vi "WriteNewCarexFile.vi"(6 "Overwrite?(F)":bool, 8 "error in (no error)":errorcluster, 9 "Proposed File Name":string, 10 "Output Path":path, 11 "CarexData In":refnum<class "CAlexData.lvclass">) -> (0 "error out":errorcluster, 1 "Actual File Name":string, 3 "CarexData Out":refnum<class "CAlexData.lvclass">)   [LabVIEW 2014, in "CAlexData.lvclass"]
uses:
  CAlexData.lvclass
  <vilib>/Utility/file.llb/Write To Spreadsheet File (string).vi
  LabView/CustomVI/CustomVI.lvlib
panel:
  out "ATIsensor":dbl[][](array[numeric])
  out "ForceComp":dbl[][](array[numeric])
  out "FieldForce":dbl[][](array[numeric])
  out "ShoulderCenter":dbl[][](array[numeric])
  out "CableLength":dbl[][](array[numeric])
  out "WaistPosition":dbl[][](array[numeric])
  out "CableTension":dbl[][](array[numeric])
  out "RefTension":dbl[][](array[numeric])
  out "JointAngle":dbl[][](array[numeric])
  out "Marker":string[](array[string])
  out "Time":dbl[](array[numeric])
  out "ExpCondition":T1
  out "ArmLength":cluster{"Upper":dbl, "Lower":dbl}
  out "FFG":T2
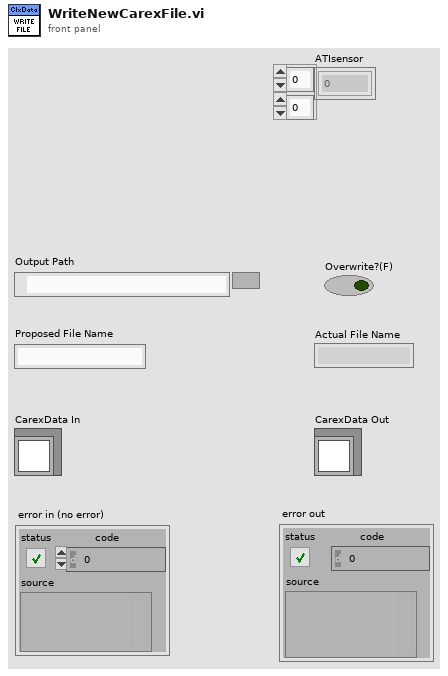
[diagram p1: front panel]
types:
  T1 = cluster{"MotorOn":bool, "EstGH":bool, "TensionMode":u16}
  T2 = cluster{"Kn":dbl, "Ns":dbl, "Kt":dbl, "Kd":dbl, "Dn":dbl, "Dt":dbl}
  T3 = enum16{"open", "replace", "create", "open or create", "replace or create", "replace or create with confirmation"}
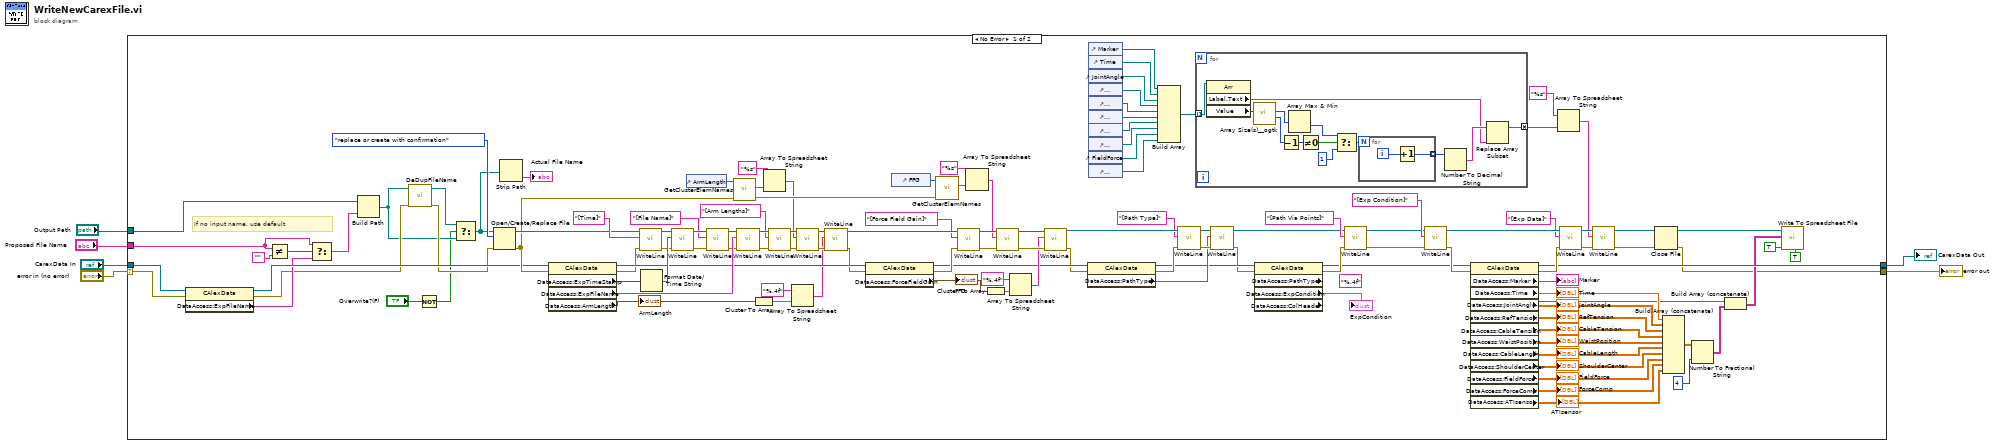
[diagram p0: block diagram]
diagram:
  n1 = case shown="No Error" "error in (no error)" {
    selector: "error in (no error)" -> [w68 w148]
    tunnel: [w73 w147] -> w5
    tunnel: [w10 w148] -> w6
    tunnel: "Output Path" -> [w60 _]
    tunnel: "CarexData In" -> [w69 w147]
    tunnel: "Proposed File Name" -> [w65 _]
    frame No Error {
      (unwired) "%.4f" ("format string")
      # "If no input name, use default"
      n2 = property class="CAlexData"(reference=w69, error in=w68) -> (reference out=w67:refnum<class "CAlexData.lvclass">, error out=w58:errorcluster, "DataAccess:ExpFileName"=w64:string)
      n3 = Not Equal?(x=w65, y="") -> (x != y?=w66:bool)
      n4 = Select(t=w65, s=w66, f=w64) -> (s? t:f=w59:string)
      n5 = Build Path(base path=w60, name or relative path=w59) -> (appended path=w56:path)
      n6 = call "DeDupFileName.vi"("error in (no error)"=w58, "Path"=w56) -> ("error out"=w57:errorcluster, "Out Path"=w63:path)  [unwired: 8 in]
      n7 = Not(x="Overwrite?(F)") -> (.not. x?=w46:bool)
      n8 = Select(t=w63, s=w46, f=w56) -> (s? t:f=w15:path)
      n9 = Open/Create/Replace File(file path (use dialog)=w15, error in=w57, operation (0:open)=T3."replace or create with confirmation") -> (refnum out=w72:refnum<file>, error out=w71:errorcluster)  [unwired: 3 in, 1 out]
      n10 = Strip Path(path=w15) -> (name=→"Actual File Name":string)  [unwired: 1 out]
      n11 = property class="CAlexData"(reference=w67, error in=w71) -> (reference out=w118:refnum<class "CAlexData.lvclass">, error out=w87:errorcluster, "DataAccess:ExpTimeStamp"=w131:timestamp, "DataAccess:ExpFileName"=w129:string, "DataAccess:ArmLength"=w119:cluster{"Upper":dbl, "Lower":dbl})
      "ArmLength" <- w119
      n12 = call "WriteLine.vi"("error in (no error)"=w87, "text"="[Time]", "refnum in"=w72) -> ("error out"=w88:errorcluster, "refnum out"=w89:refnum<file>)  [unwired: 6 in, 1 out]
      n13 = Format Date/Time String(seconds (now)=w131) -> (date/time string=w130:string)  [unwired: 2 in]
      n14 = call "WriteLine.vi"("error in (no error)"=w88, "text"=w130, "refnum in"=w89) -> ("error out"=w85:errorcluster, "refnum out"=w84:refnum<file>)  [unwired: 6 in, 1 out]
      n15 = control-ref of="ArmLength"() -> (w54:refnum<vi>)
      n16 = call "WriteLine.vi"("error in (no error)"=w85, "text"="[File Name]", "refnum in"=w84) -> ("error out"=w83:errorcluster, "refnum out"=w82:refnum<file>)  [unwired: 6 in, 1 out]
      n17 = call "GetClusterElemNames.vi"("error in (no error)"=w71, "Cluster in"=w54) -> ("error out"=w55:errorcluster, "Element Names"=w50:string[])  [unwired: 6 in, 2 out]
      n18 = call "WriteLine.vi"("error in (no error)"=w83, "text"=w129, "refnum in"=w82) -> ("error out"=w128:errorcluster, "refnum out"=w127:refnum<file>)  [unwired: 6 in, 1 out]
      n19 = Cluster To Array(cluster=w119) -> (array=w126:dbl[])
      n20 = Array To Spreadsheet String(array=w50, 3:"%s" ("format string")) -> (spreadsheet string=w49:string)  [unwired: 1 in]
      n21 = call "WriteLine.vi"("error in (no error)"=w128, "text"="[Arm Lengths]", "refnum in"=w127) -> ("error out"=w124:errorcluster, "refnum out"=w123:refnum<file>)  [unwired: 6 in, 1 out]
      n22 = Array To Spreadsheet String(array=w126, 3:"%.4f" ("format string")) -> (spreadsheet string=w117:string)  [unwired: 1 in]
      n23 = call "WriteLine.vi"("error in (no error)"=w124, "text"=w49, "refnum in"=w123) -> ("error out"=w120:errorcluster, "refnum out"=w121:refnum<file>)  [unwired: 6 in, 1 out]
      n24 = call "WriteLine.vi"("error in (no error)"=w120, "text"=w117, "refnum in"=w121) -> ("error out"=w116:errorcluster, "refnum out"=w122:refnum<file>)  [unwired: 6 in, 1 out]
      n25 = property class="CAlexData"(reference=w118, error in=w116) -> (reference out=w104:refnum<class "CAlexData.lvclass">, error out=w113:errorcluster, "DataAccess:ForceFieldGain"=w110:T2)
      "FFG" <- w110
      n26 = control-ref of="FFG"() -> (w53:refnum<vi>)
      n27 = call "GetClusterElemNames.vi"("error in (no error)"=w55, "Cluster in"=w53) -> ("Element Names"=w52:string[])  [unwired: 6 in, 3 out]
      n28 = call "WriteLine.vi"("error in (no error)"=w113, "text"="[Force Field Gain]", "refnum in"=w122) -> ("error out"=w109:errorcluster, "refnum out"=w108:refnum<file>)  [unwired: 6 in, 1 out]
      n29 = Array To Spreadsheet String(array=w52, 3:"%s" ("format string")) -> (spreadsheet string=w51:string)  [unwired: 1 in]
      n30 = Cluster To Array(cluster=w110) -> (array=w111:dbl[])
      n31 = call "WriteLine.vi"("error in (no error)"=w109, "text"=w51, "refnum in"=w108) -> ("error out"=w107:errorcluster, "refnum out"=w106:refnum<file>)  [unwired: 6 in, 1 out]
      n32 = Array To Spreadsheet String(array=w111, 3:"%.4f" ("format string")) -> (spreadsheet string=w105:string)  [unwired: 1 in]
      n33 = call "WriteLine.vi"("error in (no error)"=w107, "text"=w105, "refnum in"=w106) -> ("error out"=w103:errorcluster, "refnum out"=w102:refnum<file>)  [unwired: 6 in, 1 out]
      n34 = property class="CAlexData"(reference=w104, error in=w103) -> (reference out=w93:refnum<class "CAlexData.lvclass">, error out=w101:errorcluster, "DataAccess:PathType"=w98:string)
      n35 = control-ref of="Marker"() -> (w43:refnum<vi>)
      n36 = control-ref of="Time"() -> (w42:refnum<vi>)
      n37 = control-ref of="JointAngle"() -> (w41:refnum<vi>)
      n38 = control-ref of="RefTension"() -> (w40:refnum<vi>)
      n39 = control-ref of="CableTension"() -> (w39:refnum<vi>)
      n40 = control-ref of="WaistPosition"() -> (w38:refnum<vi>)
      n41 = control-ref of="CableLength"() -> (w37:refnum<vi>)
      n42 = control-ref of="ShoulderCenter"() -> (w36:refnum<vi>)
      n43 = control-ref of="FieldForce"() -> (w35:refnum<vi>)
      n44 = control-ref of="ForceComp"() -> (w34:refnum<vi>)
      n45 = Build Array(w43, w42, w41, w40, w39, w38, w37, w36, w35, w34) -> (w33:refnum<vi>[])
      n46 = call "WriteLine.vi"("error in (no error)"=w101, "text"="[Path Type]", "refnum in"=w102) -> ("error out"=w100:errorcluster, "refnum out"=w99:refnum<file>)  [unwired: 6 in, 1 out]
      n47 = for {
        tunnel: w33 -> [w144] mode=indexing
        tunnel: [w140] -> w17 mode=concatenating
        n48 = property class="Arr"(reference=w144) -> ("Label.Text"=w141:string, "Value"=w139:variant)  [unwired: 1 in, 2 out]
        n49 = call <userlib>:"Array Size(s)__ogtk.vi"("Array"=w139) -> ("N dims"=w137:u32, "Size(s)"=w138:u32[])  [unwired: 8 in, 1 out]
        n50 = Decrement(x=w137) -> (x-1=w136:u32)
        n51 = Array Max & Min(array=w138) -> (min value=w132:u32)  [unwired: 3 out]
        n52 = Not Equal To 0?(x=w136) -> (x != 0?=w134:bool)
        n53 = Select(t=w132, s=w134, f=u32 1) -> (s? t:f=w135:u32)
        n54 = for {
          N: w135 -> [_]
          tunnel: [w145] -> w143 mode=indexing
          i -> [w146]
          n55 = Increment(x=w146) -> (x+1=w145:i32)
        }
        n56 = Number To Decimal String(number=w143) -> (decimal integer string=w142:string[])  [unwired: 1 in]
        n57 = Replace Array Subset(array=w142, new element=w141) -> (w140:string[])  [unwired: 1 in]
      }
      n58 = call "WriteLine.vi"("error in (no error)"=w100, "text"=w98, "refnum in"=w99) -> ("error out"=w92:errorcluster, "refnum out"=w94:refnum<file>)  [unwired: 6 in, 1 out]
      n59 = property class="CAlexData" props=["DataAccess:PathType", "DataAccess:ExpCondition", "DataAccess:ColHeader"](reference=w93, error in=w92) -> (reference out=w79:refnum<class "CAlexData.lvclass">, error out=w95:errorcluster, "DataAccess:ExpCondition"=→"ExpCondition":T1)  [unwired: 2 out]
      n60 = call "WriteLine.vi"("error in (no error)"=w95, "text"="[Path Via Points]", "refnum in"=w94) -> ("error out"=w7:errorcluster, "refnum out"=w8:refnum<file>)  [unwired: 6 in, 1 out]
      n61 = call "WriteLine.vi"("error in (no error)"=w7, "text"="[Exp Condition]", "refnum in"=w8) -> ("error out"=w80:errorcluster, "refnum out"=w78:refnum<file>)  [unwired: 6 in, 1 out]
      n62 = property class="CAlexData"(reference=w79, error in=w80) -> (reference out=w73:refnum<class "CAlexData.lvclass">, error out=w77:errorcluster, "DataAccess:Marker"=w19:string[], "DataAccess:Time"=w30:dbl[], "DataAccess:JointAngle"=w29:dbl[][], "DataAccess:RefTension"=w28:dbl[][], "DataAccess:CableTension"=w27:dbl[][], "DataAccess:WaistPosition"=w26:dbl[][], "DataAccess:CableLength"=w25:dbl[][], "DataAccess:ShoulderCenter"=w24:dbl[][], "DataAccess:FieldForce"=w23:dbl[][], "DataAccess:ForceComp"=w22:dbl[][], "DataAccess:ATIsensor"=w9:dbl[][])
      "Time" <- w30
      "Marker" <- w19
      "JointAngle" <- w29
      "RefTension" <- w28
      "CableTension" <- w27
      "WaistPosition" <- w26
      "CableLength" <- w25
      "ShoulderCenter" <- w24
      "FieldForce" <- w23
      "ForceComp" <- w22
      "ATIsensor" <- w9
      n63 = Array To Spreadsheet String(array=w17, 3:"%s" ("format string")) -> (spreadsheet string=w32:string)  [unwired: 1 in]
      n64 = call "WriteLine.vi"("error in (no error)"=w77, "text"="[Exp Data]", "refnum in"=w78) -> ("error out"=w75:errorcluster, "refnum out"=w74:refnum<file>)  [unwired: 6 in, 1 out]
      n65 = call "WriteLine.vi"("error in (no error)"=w75, "text"=w32, "refnum in"=w74) -> ("error out"=w11:errorcluster, "refnum out"=w13:refnum<file>)  [unwired: 6 in, 1 out]
      n66 = Close File(refnum=w13, error in=w11) -> (path=w12:path, error out=w10:errorcluster)
      n67 = Build Array (concatenate)(w30, w29, w28, w27, w26, w25, w24, w23, w22, w9) -> (w21:dbl[][])
      n68 = Number To Fractional String(number=w21, precision (6)=i16 4) -> (F-format string=w20:string[][])  [unwired: 2 in]
      n69 = Build Array (concatenate)(w19, w20) -> (w18:string[][])
      n70 = call-poly <vilib>:"Write To Spreadsheet File.vi"("transpose? (no:F)"=TRUE, "append to file? (new file:F)"=TRUE, "2D data"=w18, "file path (dialog if empty)"=w12) -> ()  [unwired: 4 in, 1 out]
    }
    frame Error {
    }
  }
  "CarexData Out" <- w5
  "error out" <- w6
